vi "Configure External Out Trigger.vi"(7 "Logic Type (1: Negative)":i32(ring)=1 items=["Positive", "Negative"], 8 "error in (no error)":errorcluster, 9 "External Stimulus Event (\"NONE\")":string="NONE", 11 "VISA resource name":refnum<visa-resource-name>) -> (0 "error out":errorcluster, 3 "VISA resource name out":refnum<visa-resource-name>)   [LabVIEW 2015, in "Keithley DMM6500 DAQ6500 Series.lvlib"]
doc: "Sets the output logic of the trigger event generator to positive or negative for the TRIGGER OUT line and selects the event that causes a trigger to be asserted on the TRIGGER OUT line."
uses:
  <instrlib>/Keithley DMM6500 DAQ6500 Series/Keithley DMM6500 DAQ6500 Series.lvlib
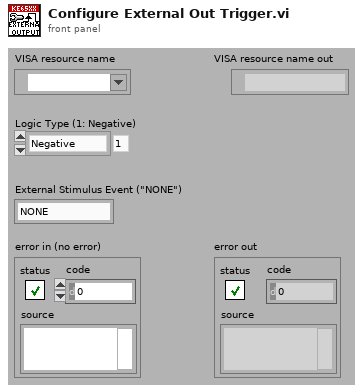
[diagram p1: front panel]
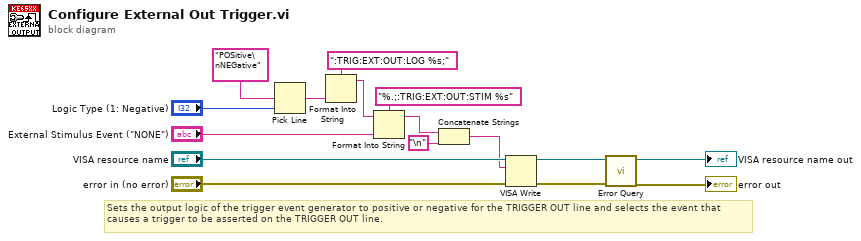
[diagram p0: block diagram]
diagram:
  # "Sets the output logic of the trigger event generator to positive or negative for the TRIGGER OUT line and selects the event that causes a trigger to be asserted on the TRIGGER OUT line."
  n1 = Pick Line(multi-line string="POSitive\nNEGative", line index="Logic Type (1: Negative)") -> (output string=w4:string)  [unwired: 1 in]
  n2 = Format Into String(format string=":TRIG:EXT:OUT:LOG %s;", w4) -> (resulting string=w15:string)  [unwired: 2 in, 1 out]
  n3 = Format Into String(format string="%.;:TRIG:EXT:OUT:STIM %s", initial string=w15, "External Stimulus Event (\"NONE\")") -> (resulting string=w1:string)  [unwired: 1 in, 1 out]
  n4 = Concatenate Strings(w1, "\n") -> (w3:string)
  n5 = VISA Write(VISA resource name="VISA resource name", write buffer=w3, error in (no error)="error in (no error)") -> (VISA resource name out=w10:refnum<visa-resource-name>, error out=w9:errorcluster)  [unwired: 1 out]
  n6 = call <instrlib>:"Error Query.vi"("error in (no error)"=w9, "VISA resource name"=w10) -> ("error out"=→"error out":errorcluster, "VISA resource name out"=→"VISA resource name out":refnum<visa-resource-name>)  [unwired: 6 in, 2 out]
